vi "Descarga_VFD.vi"(5 "Fabricante":u32, 6 "Modbus":T4, 7 "Iteraciones (In)":u32, 8 "Motor":T6, 9 "I/O":T7, 10 "Referencias":T5, 11 "Instancia Modbus":refnum<class "Modbus Master.lvclass">) -> (0 "Error Modbus":errorcluster, 2 "Iteraciones (Out)":u32)   [LabVIEW 2013]
uses:
  <vilib>/NI/Modbus Library/API/Master/Modbus Master.lvclass
panel:
  in  "Modbus ACS-180":T1
  in  "Modbus VFD-EL":T2
  in  "Modbus ATV 320":T3
  in  "M ACS-180":T1
  in  "M VFD-EL":T2
  in  "M ATV 320":T3
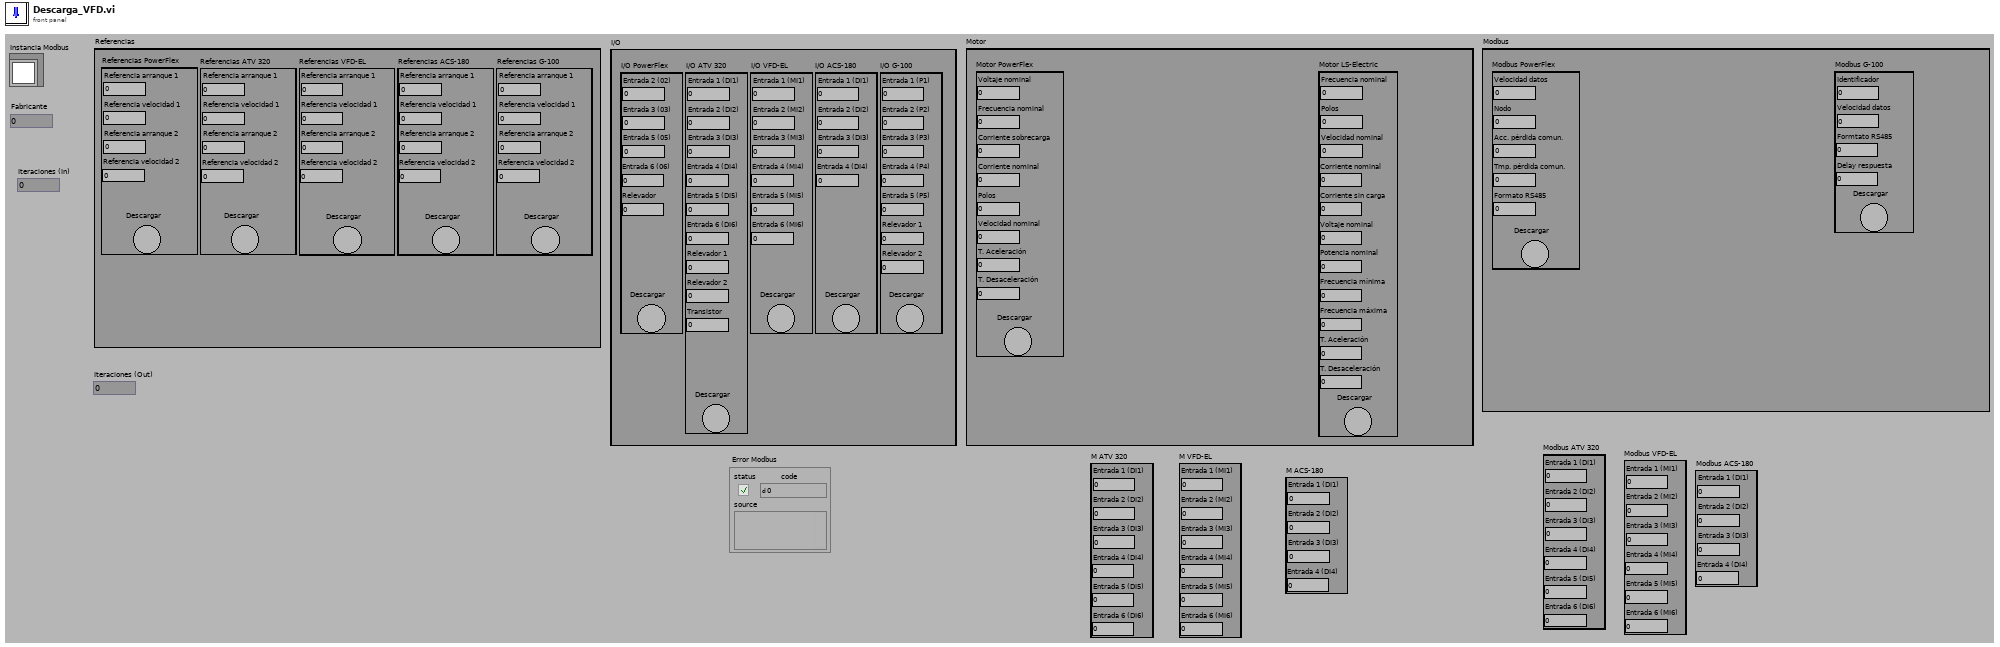
[diagram p1: front panel]
types:
  T1 = cluster{"Entrada 1 (DI1)":u16, "Entrada 2 (DI2)":u16, "Entrada 3 (DI3)":u16, "Entrada 4 (DI4)":u16}
  T2 = cluster{"Entrada 1 (MI1)":u16, "Entrada 2 (MI2)":u16, "Entrada 3 (MI3)":u16, "Entrada 4 (MI4)":u16, "Entrada 5 (MI5)":u16, "Entrada 6 (MI6)":u16}
  T3 = cluster{"Entrada 1 (DI1)":u16, "Entrada 2 (DI2)":u16, "Entrada 3 (DI3)":u16, "Entrada 4 (DI4)":u16, "Entrada 5 (DI5)":u16, "Entrada 6 (DI6)":u16}
  T4 = cluster{"Modbus PowerFlex":cluster{"Velocidad datos":u16, "Nodo":u16, "Acc. pérdida comun.":u16, "Tmp. pérdida comun.":u16, "Formato RS485":u16, "Descargar":bool}, "Modbus G-100":cluster{"Identificador":u16, "Velocidad datos":u16, "Formtato RS485":u16, "Delay respuesta":u16, "Descargar":bool}}
  T5 = cluster{"Referencias PowerFlex":cluster{"Referencia arranque 1":u16, "Referencia velocidad 1":u16, "Referencia arranque 2":u16, "Referencia velocidad 2":u16, "Descargar":bool}, "Referencias ATV 320":cluster{"Referencia arranque 1":u16, "Referencia velocidad 1":u16, "Referencia arranque 2":u16, "Referencia velocidad 2":u16, "Descargar":bool}, "Referencias VFD-EL":cluster{"Referencia arranque 1":u16, "Referencia velocidad 1":u16, "Referencia arranque 2":u16, "Referencia velocidad 2":u16, "Descargar":bool}, "Referencias ACS-180":cluster{"Referencia arranque 1":u16, "Referencia velocidad 1":u16, "Referencia arranque 2":u16, "Referencia velocidad 2":u16, "Descargar":bool}, "Referencias G-100":cluster{"Referencia arranque 1":u16, "Referencia velocidad 1":u16, "Referencia arranque 2":u16, "Referencia velocidad 2":u16, "Descargar":bool}}
  T6 = cluster{"Motor PowerFlex":cluster{"Voltaje nominal":u16, "Frecuencia nominal":u16, "Corriente sobrecarga":dbl, "Corriente nominal":dbl, "Polos":u16, "Velocidad nominal":u16, "T. Aceleración":dbl, "T. Desaceleración":dbl, "Descargar":bool}, "Motor LS-Electric":cluster{"Frecuencia nominal":u16, "Polos":u16, "Velocidad nominal":u16, "Corriente nominal":dbl, "Corriente sin carga":dbl, "Voltaje nominal":u16, "Potencia nominal":u16, "Frecuencia mínima":dbl, "Frecuencia máxima":dbl, "T. Aceleración":dbl, "T. Desaceleración":dbl, "Descargar":bool}}
  T7 = cluster{"I/O PowerFlex":cluster{"Entrada 2 (02)":u16, "Entrada 3 (03)":u16, "Entrada 5 (05)":u16, "Entrada 6 (06)":u16, "Relevador":u16, "Descargar":bool}, "I/O ATV 320":cluster{"Entrada 1 (DI1)":u16, "Entrada 2 (DI2)":u16, "Entrada 3 (DI3)":u16, "Entrada 4 (DI4)":u16, "Entrada 5 (DI5)":u16, "Entrada 6 (DI6)":u16, "Relevador 1":u16, "Relevador 2":u16, "Transistor":u16, "Descargar":bool}, "I/O VFD-EL":cluster{"Entrada 1 (MI1)":u16, "Entrada 2 (MI2)":u16, "Entrada 3 (MI3)":u16, "Entrada 4 (MI4)":u16, "Entrada 5 (MI5)":u16, "Entrada 6 (MI6)":u16, "Descargar":bool}, "I/O ACS-180":cluster{"Entrada 1 (DI1)":u16, "Entrada 2 (DI2)":u16, "Entrada 3 (DI3)":u16, "Entrada 4 (DI4)":u16, "Descargar":bool}, "I/O G-100":cluster{"Entrada 1 (P1)":u16, "Entrada 2 (P2)":u16, "Entrada 3 (P3)":u16, "Entrada 4 (P4)":u16, "Entrada 5 (P5)":u16, "Relevador 1":u16, "Relevador 2":u16, "Descargar":bool}}
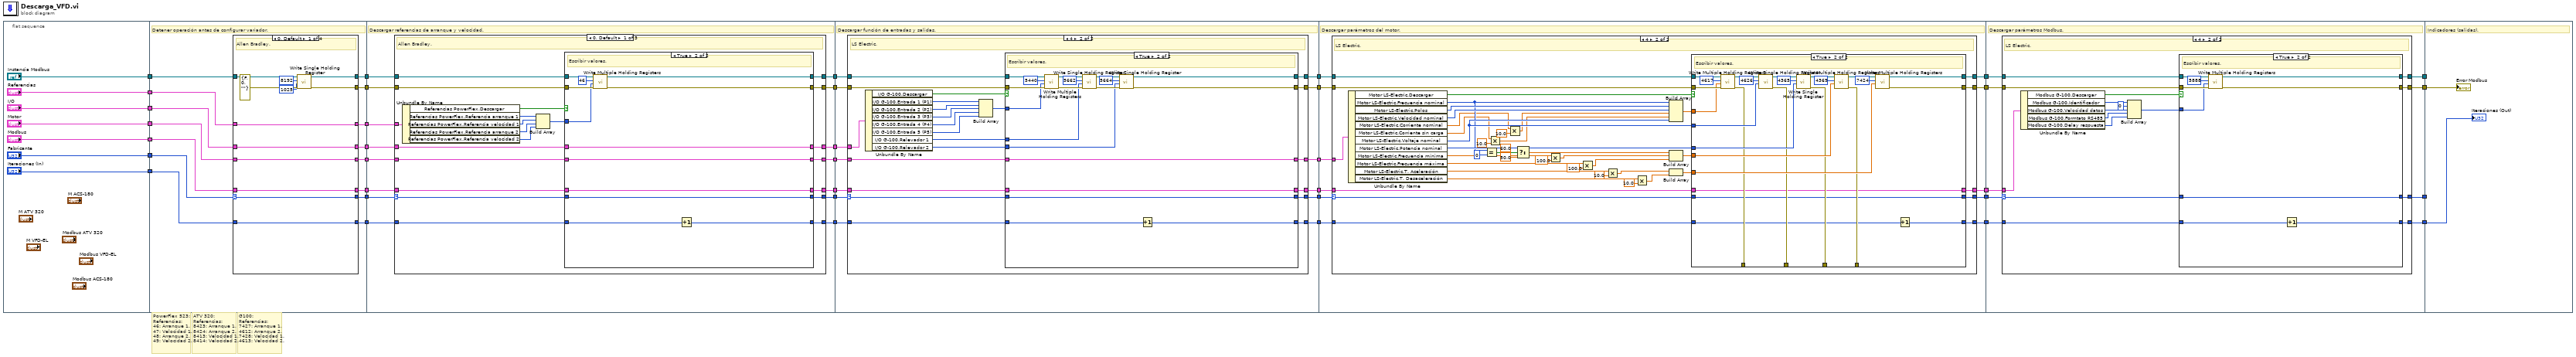
[diagram p0: block diagram]
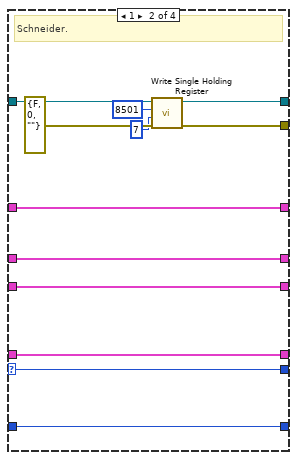
[diagram p2: hidden frame]
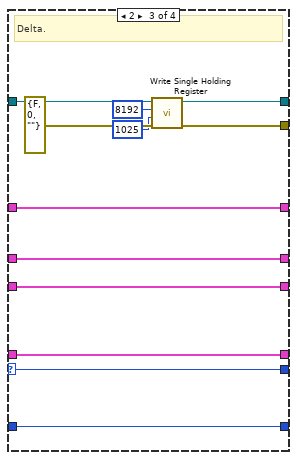
[diagram p3: hidden frame]
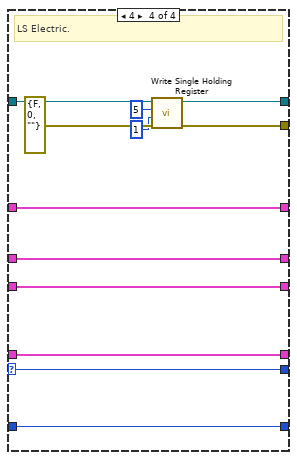
[diagram p4: hidden frame]
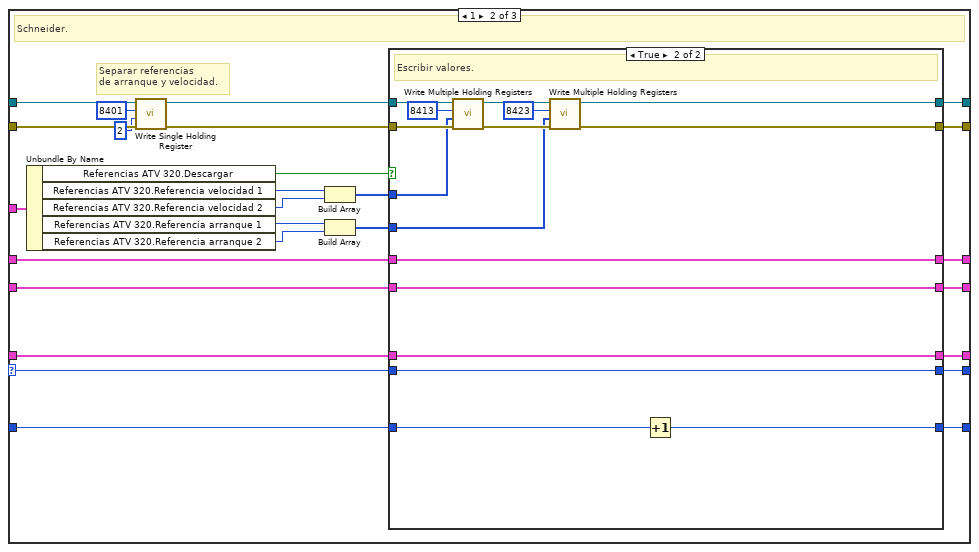
[diagram p6: hidden frame]
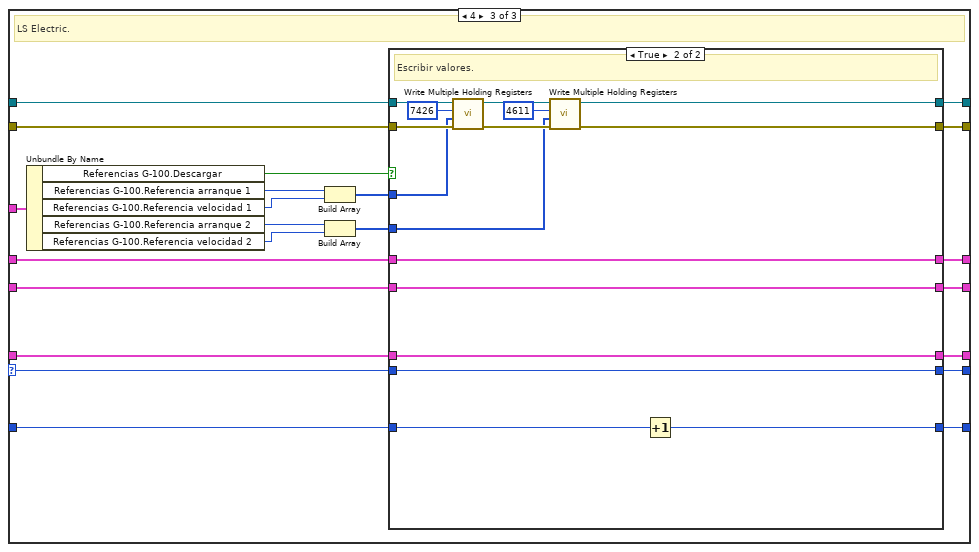
[diagram p8: hidden frame]
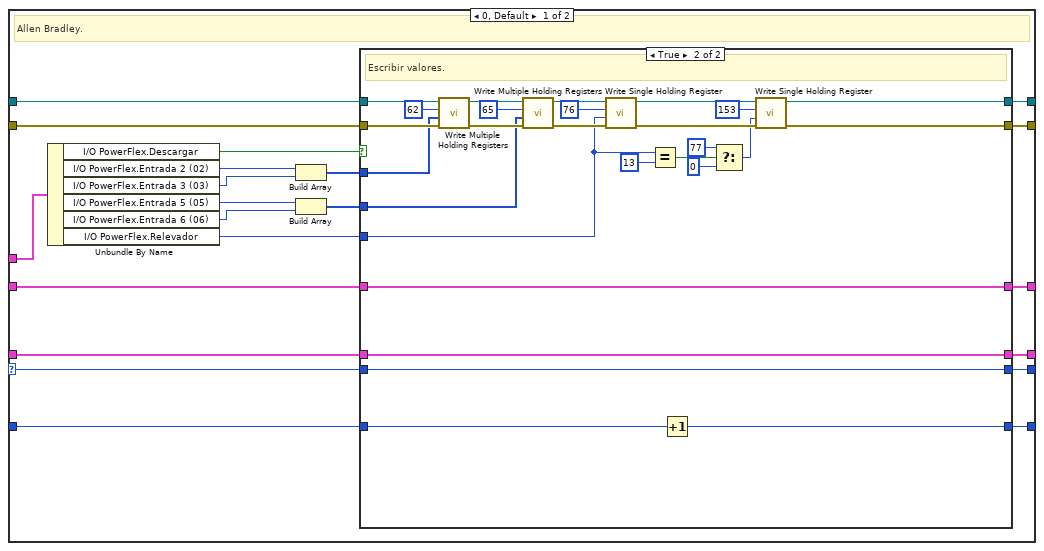
[diagram p10: hidden frame]
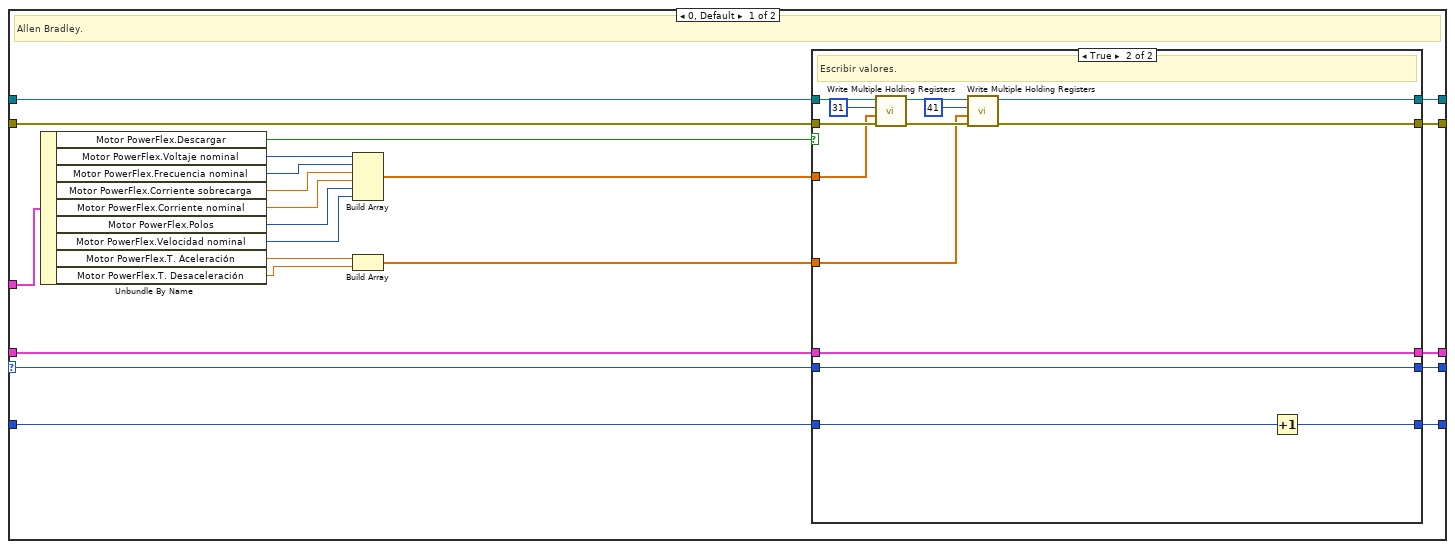
[diagram p13: hidden frame]
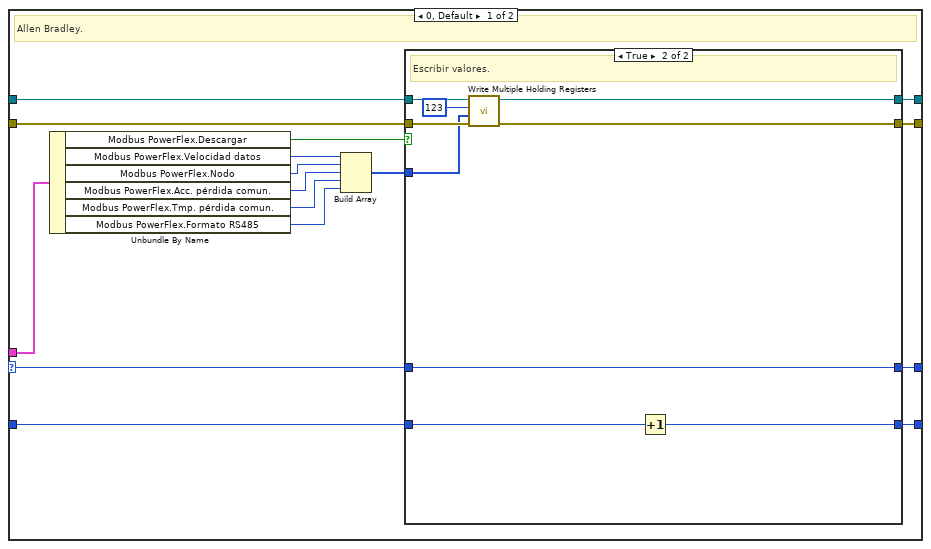
[diagram p16: hidden frame]
diagram:
  # "G100:\nReferencias:\n7427: Arranque 1.\n4612: Arranque 2.\n7428: Velocidad 1.\n4613: Velocidad 2."
  # "ATV 320:\nReferencias:\n8423: Arranque 1.\n8424: Arranque 2.\n8413: Velocidad 1.\n8414: Velocidad 2."
  # "PowerFlex 523:\nReferencias:\n46: Arranque 1.\n47: Velocidad 1.\n48: Arranque 2.\n49: Velocidad 2."
  n1 = flat-sequence {
    tunnel: ["Instancia Modbus"] -> w34
    tunnel: ["Fabricante"] -> w32
    tunnel: ["Referencias"] -> w31
    tunnel: ["I/O"] -> w27
    tunnel: ["Motor"] -> w21
    tunnel: ["Iteraciones (In)"] -> w17
    tunnel: ["Modbus"] -> w13
    tunnel: w34 -> [w59]
    tunnel: [w58] -> w33
    tunnel: w32 -> [w56]
    tunnel: w31 -> [w54]
    tunnel: [w53] -> w30
    tunnel: [w57] -> w29
    tunnel: [w55] -> w28
    tunnel: w27 -> [w52]
    tunnel: [w51] -> w26
    tunnel: w21 -> [w50]
    tunnel: [w49] -> w20
    tunnel: w17 -> [w48]
    tunnel: [w47] -> w16
    tunnel: w13 -> [w46]
    tunnel: [w45] -> w12
    tunnel: w33 -> [w122]
    tunnel: w30 -> [w120]
    tunnel: [w121] -> w37
    tunnel: [w119] -> w36
    tunnel: [w118] -> w35
    tunnel: w29 -> [w117]
    tunnel: w28 -> [w116]
    tunnel: w26 -> [w115]
    tunnel: [w114] -> w25
    tunnel: w20 -> [w113]
    tunnel: [w112] -> w19
    tunnel: w16 -> [w111]
    tunnel: [w110] -> w15
    tunnel: w12 -> [w109]
    tunnel: [w108] -> w11
    tunnel: w37 -> [w268]
    tunnel: w36 -> [w267]
    tunnel: w35 -> [w269]
    tunnel: w25 -> [w266]
    tunnel: [w265] -> w24
    tunnel: [w264] -> w23
    tunnel: [w263] -> w22
    tunnel: w19 -> [w262]
    tunnel: [w261] -> w18
    tunnel: w15 -> [w260]
    tunnel: [w259] -> w14
    tunnel: w11 -> [w258]
    tunnel: [w257] -> w10
    tunnel: w24 -> [w380]
    tunnel: w23 -> [w379]
    tunnel: w22 -> [w381]
    tunnel: w18 -> [w378]
    tunnel: w14 -> [w377]
    tunnel: w10 -> [w376]
    tunnel: [w375] -> w9
    tunnel: [w374] -> w8
    tunnel: [w373] -> w7
    tunnel: [w372] -> w6
    tunnel: [w371] -> w5
    tunnel: w9 -> [w505]
    tunnel: w8 -> [w504]
    tunnel: w7 -> [w501]
    tunnel: w6 -> [w503]
    tunnel: w5 -> [w502]
    tunnel: [w500] -> w4
    tunnel: [w499] -> w3
    tunnel: [w498] -> w2
    tunnel: [w497] -> w1
    tunnel: w4 -> [w565]
    tunnel: w3 -> [_]
    tunnel: w2 -> [w564]
    tunnel: w1 -> [_]
    frame #0 {
    }
    frame #1 {
      # "Detener operación antes de configurar variador."
      n2 = case shown="0, Default" w56 {
        selector: w56 -> [w70 w82 w94 w106]
        tunnel: w59 -> [w67 w79 w91 w103]
        tunnel: [w65 w77 w89 w101] -> w58
        tunnel: [w66 w78 w90 w102] -> w57
        tunnel: [w70 w82 w94 w106] -> w55
        tunnel: w54 -> [w64 w76 w88 w100]
        tunnel: [w64 w76 w88 w100] -> w53
        tunnel: w52 -> [w63 w75 w87 w99]
        tunnel: [w63 w75 w87 w99] -> w51
        tunnel: w50 -> [w62 w74 w86 w98]
        tunnel: [w62 w74 w86 w98] -> w49
        tunnel: w48 -> [w61 w73 w85 w97]
        tunnel: [w61 w73 w85 w97] -> w47
        tunnel: w46 -> [w60 w72 w84 w96]
        tunnel: [w60 w72 w84 w96] -> w45
        frame 0, Default {
          # "Allen Bradley."
          n3 = call-dynamic "Write Single Holding Register.vi"("error in"=errorcluster {"status"=FALSE, "code"=0, "source"=""}, "register to write"=u16 1025, "address"=u16 8192, "Modbus master in"=w67) -> ("error out"=w66:errorcluster, "Modbus master out"=w65:refnum<class "Modbus Master.lvclass">)  [unwired: 6 in]
        }
        frame 1 {
          # "Schneider."
          n4 = call-dynamic "Write Single Holding Register.vi"("error in"=errorcluster {"status"=FALSE, "code"=0, "source"=""}, "register to write"=u16 7, "address"=u16 8501, "Modbus master in"=w79) -> ("error out"=w78:errorcluster, "Modbus master out"=w77:refnum<class "Modbus Master.lvclass">)  [unwired: 6 in]
        }
        frame 2 {
          # "Delta."
          n5 = call-dynamic "Write Single Holding Register.vi"("error in"=errorcluster {"status"=FALSE, "code"=0, "source"=""}, "register to write"=u16 1025, "address"=u16 8192, "Modbus master in"=w91) -> ("error out"=w90:errorcluster, "Modbus master out"=w89:refnum<class "Modbus Master.lvclass">)  [unwired: 6 in]
        }
        frame 4 {
          # "LS Electric."
          n6 = call-dynamic "Write Single Holding Register.vi"("error in"=errorcluster {"status"=FALSE, "code"=0, "source"=""}, "register to write"=u16 1, "address"=u16 5, "Modbus master in"=w103) -> ("error out"=w102:errorcluster, "Modbus master out"=w101:refnum<class "Modbus Master.lvclass">)  [unwired: 6 in]
        }
      }
    }
    frame #2 {
      # "Descargar referencias de arranque y velocidad."
      n7 = case shown="0, Default" w116 {
        selector: w116 -> [w129 w169 w215]
        tunnel: w122 -> [w139 w183 w232]
        tunnel: [w142 w185 w229] -> w121
        tunnel: w120 -> [w141 w186 w230]
        tunnel: [w140 w184 w228] -> w119
        tunnel: [w124 w164 w214] -> w118
        tunnel: w117 -> [w143 w188 w233]
        tunnel: w115 -> [w132 w172 w221]
        tunnel: [w127 w167 w220] -> w114
        tunnel: w113 -> [w131 w171 w219]
        tunnel: [w126 w166 w218] -> w112
        tunnel: w111 -> [w128 w168 w213]
        tunnel: [w123 w163 w212] -> w110
        tunnel: w109 -> [w130 w170 w217]
        tunnel: [w125 w165 w216] -> w108
        frame 0, Default {
          # "Allen Bradley."
          n8 = Unbundle By Name(w141) -> ("Referencias PowerFlex.Descargar"=w133:bool, "Referencias PowerFlex.Referencia arranque 1"=w137:u16, "Referencias PowerFlex.Referencia velocidad 1"=w136:u16, "Referencias PowerFlex.Referencia arranque 2"=w135:u16, "Referencias PowerFlex.Referencia velocidad 2"=w134:u16)
          n9 = Build Array(w137, w136, w135, w134) -> (w138:u16[])
          n10 = case shown="True" w133 {
            tunnel: w143 -> [w149 w162]
            tunnel: [w150 w161] -> w142
            tunnel: [w149 w159] -> w140
            tunnel: w139 -> [w150 w158]
            tunnel: w138 -> [_ w157]
            tunnel: w132 -> [w148 w156]
            tunnel: w131 -> [w147 w155]
            tunnel: w130 -> [w146 w154]
            tunnel: w129 -> [w145 w153]
            tunnel: w128 -> [w144 w152]
            tunnel: [w148 w156] -> w127
            tunnel: [w147 w155] -> w126
            tunnel: [w146 w154] -> w125
            tunnel: [w145 w153] -> w124
            tunnel: [w144 w151] -> w123
            frame False {
              # "Nada."
            }
            frame True {
              # "Escribir valores."
              n11 = call-dynamic "Write Multiple Holding Registers.vi"("error in"=w162, "registers to write"=w157, "starting address"=u16 46, "Modbus master in"=w158) -> ("error out"=w159:errorcluster, "Modbus master out"=w161:refnum<class "Modbus Master.lvclass">)  [unwired: 6 in]
              n12 = Increment(x=w152) -> (x+1=w151:u32)
            }
          }
        }
        frame 1 {
          # "Separar referencias\nde arranque y velocidad."
          # "Schneider."
          n13 = Unbundle By Name(w186) -> ("Referencias ATV 320.Descargar"=w177:bool, "Referencias ATV 320.Referencia velocidad 1"=w176:u16, "Referencias ATV 320.Referencia velocidad 2"=w175:u16, "Referencias ATV 320.Referencia arranque 1"=w174:u16, "Referencias ATV 320.Referencia arranque 2"=w173:u16)
          n14 = call-dynamic "Write Single Holding Register.vi"("error in"=w188, "register to write"=u16 2, "address"=u16 8401, "Modbus master in"=w183) -> ("error out"=w187:errorcluster, "Modbus master out"=w182:refnum<class "Modbus Master.lvclass">)  [unwired: 6 in]
          n15 = Build Array(w176, w175) -> (w179:u16[])
          n16 = Build Array(w174, w173) -> (w178:u16[])
          n17 = case shown="True" w177 {
            tunnel: w187 -> [w194 w211]
            tunnel: [w195 w207] -> w185
            tunnel: [w194 w206] -> w184
            tunnel: w182 -> [w195 w204]
            tunnel: w179 -> [_ w203]
            tunnel: w178 -> [_ w202]
            tunnel: w172 -> [w193 w201]
            tunnel: w171 -> [w192 w200]
            tunnel: w170 -> [w191 w199]
            tunnel: w169 -> [w190 w198]
            tunnel: w168 -> [w189 w197]
            tunnel: [w193 w201] -> w167
            tunnel: [w192 w200] -> w166
            tunnel: [w191 w199] -> w165
            tunnel: [w190 w198] -> w164
            tunnel: [w189 w196] -> w163
            frame False {
              # "Nada."
            }
            frame True {
              # "Escribir valores."
              n18 = call-dynamic "Write Multiple Holding Registers.vi"("error in"=w211, "registers to write"=w203, "starting address"=u16 8413, "Modbus master in"=w204) -> ("error out"=w205:errorcluster, "Modbus master out"=w208:refnum<class "Modbus Master.lvclass">)  [unwired: 6 in]
              n19 = call-dynamic "Write Multiple Holding Registers.vi"("error in"=w205, "registers to write"=w202, "starting address"=u16 8423, "Modbus master in"=w208) -> ("error out"=w206:errorcluster, "Modbus master out"=w207:refnum<class "Modbus Master.lvclass">)  [unwired: 6 in]
              n20 = Increment(x=w197) -> (x+1=w196:u32)
            }
          }
        }
        frame 4 {
          # "LS Electric."
          n21 = Unbundle By Name(w230) -> ("Referencias G-100.Descargar"=w226:bool, "Referencias G-100.Referencia arranque 1"=w225:u16, "Referencias G-100.Referencia velocidad 1"=w224:u16, "Referencias G-100.Referencia arranque 2"=w223:u16, "Referencias G-100.Referencia velocidad 2"=w222:u16)
          n22 = Build Array(w225, w224) -> (w231:u16[])
          n23 = Build Array(w223, w222) -> (w227:u16[])
          n24 = case shown="True" w226 {
            tunnel: w233 -> [w239 w256]
            tunnel: w232 -> [w240 w255]
            tunnel: w231 -> [_ w253]
            tunnel: [w240 w250] -> w229
            tunnel: [w239 w249] -> w228
            tunnel: w227 -> [_ w247]
            tunnel: w221 -> [w238 w246]
            tunnel: [w238 w246] -> w220
            tunnel: w219 -> [w237 w245]
            tunnel: [w237 w245] -> w218
            tunnel: w217 -> [w236 w244]
            tunnel: [w236 w244] -> w216
            tunnel: [w235 w243] -> w214
            tunnel: w215 -> [w235 w243]
            tunnel: w213 -> [w234 w242]
            tunnel: [w234 w241] -> w212
            frame False {
              # "Nada."
            }
            frame True {
              # "Escribir valores."
              n25 = call-dynamic "Write Multiple Holding Registers.vi"("error in"=w256, "registers to write"=w253, "starting address"=u16 7426, "Modbus master in"=w255) -> ("error out"=w248:errorcluster, "Modbus master out"=w251:refnum<class "Modbus Master.lvclass">)  [unwired: 6 in]
              n26 = call-dynamic "Write Multiple Holding Registers.vi"("error in"=w248, "registers to write"=w247, "starting address"=u16 4611, "Modbus master in"=w251) -> ("error out"=w249:errorcluster, "Modbus master out"=w250:refnum<class "Modbus Master.lvclass">)  [unwired: 6 in]
              n27 = Increment(x=w242) -> (x+1=w241:u32)
            }
          }
        }
      }
    }
    frame #3 {
      # "Descargar función de entradas y salidas."
      n28 = case shown="4" w269 {
        selector: w269 -> [w275 w329]
        tunnel: w268 -> [w288 w342]
        tunnel: [w271 w325] -> w263
        tunnel: w267 -> [w289 w343]
        tunnel: w266 -> [w290 w344]
        tunnel: [w285 w340] -> w265
        tunnel: [w284 w339] -> w264
        tunnel: w262 -> [w277 w331]
        tunnel: [w273 w327] -> w261
        tunnel: w260 -> [w274 w328]
        tunnel: [w270 w324] -> w259
        tunnel: w258 -> [w276 w330]
        tunnel: [w272 w326] -> w257
        frame 0, Default {
          # "Allen Bradley."
          n29 = Unbundle By Name(w290) -> ("I/O PowerFlex.Descargar"=w278:bool, "I/O PowerFlex.Entrada 2 (02)"=w282:u16, "I/O PowerFlex.Entrada 3 (03)"=w281:u16, "I/O PowerFlex.Entrada 5 (05)"=w280:u16, "I/O PowerFlex.Entrada 6 (06)"=w279:u16, "I/O PowerFlex.Relevador"=w283:u16)
          n30 = Build Array(w282, w281) -> (w287:u16[])
          n31 = Build Array(w280, w279) -> (w286:u16[])
          n32 = case shown="True" w278 {
            tunnel: w289 -> [w295 w322]
            tunnel: w288 -> [w296 w321]
            tunnel: w287 -> [_ w319]
            tunnel: w286 -> [_ w315]
            tunnel: [w296 w304] -> w285
            tunnel: [w295 w303] -> w284
            tunnel: w283 -> [_ w302]
            tunnel: w277 -> [w294 w301]
            tunnel: w276 -> [w293 w300]
            tunnel: w275 -> [w292 w299]
            tunnel: w274 -> [w291 w298]
            tunnel: [w294 w301] -> w273
            tunnel: [w293 w300] -> w272
            tunnel: [w292 w299] -> w271
            tunnel: [w291 w297] -> w270
            frame False {
              # "Nada."
            }
            frame True {
              # "Escribir valores."
              n33 = call-dynamic "Write Multiple Holding Registers.vi"("error in"=w322, "registers to write"=w319, "starting address"=u16 62, "Modbus master in"=w321) -> ("error out"=w316:errorcluster, "Modbus master out"=w317:refnum<class "Modbus Master.lvclass">)  [unwired: 6 in]
              n34 = call-dynamic "Write Multiple Holding Registers.vi"("error in"=w316, "registers to write"=w315, "starting address"=u16 65, "Modbus master in"=w317) -> ("error out"=w323:errorcluster, "Modbus master out"=w313:refnum<class "Modbus Master.lvclass">)  [unwired: 6 in]
              n35 = call-dynamic "Write Single Holding Register.vi"("error in"=w323, "register to write"=w302, "address"=u16 76 ("starting address"), "Modbus master in"=w313) -> ("error out"=w311:errorcluster, "Modbus master out"=w310:refnum<class "Modbus Master.lvclass">)  [unwired: 6 in]
              n36 = Equal?(x=w302, y=u16 13) -> (x = y?=w308:bool)
              n37 = Increment(x=w298) -> (x+1=w297:u32)
              n38 = Select(t=u16 77 ("register to write"), s=w308, f=u16 0 ("register to write")) -> (s? t:f=w305:u16)
              n39 = call-dynamic "Write Single Holding Register.vi"("error in"=w311, "register to write"=w305, "address"=u16 153 ("starting address"), "Modbus master in"=w310) -> ("error out"=w303:errorcluster, "Modbus master out"=w304:refnum<class "Modbus Master.lvclass">)  [unwired: 6 in]
            }
          }
        }
        frame 4 {
          # "LS Electric."
          n40 = Unbundle By Name(w344) -> ("I/O G-100.Descargar"=w335:bool, "I/O G-100.Entrada 1 (P1)"=w333:u16, "I/O G-100.Entrada 2 (P2)"=w332:u16, "I/O G-100.Entrada 3 (P3)"=w338:u16, "I/O G-100.Entrada 4 (P4)"=w337:u16, "I/O G-100.Entrada 5 (P5)"=w336:u16, "I/O G-100.Relevador 1"=w345:u16, "I/O G-100.Relevador 2"=w334:u16)
          n41 = Build Array(w333, w332, w338, w337, w336) -> (w341:u16[])
          n42 = case shown="True" w335 {
            tunnel: w345 -> [_ w358]
            tunnel: w343 -> [w350 w368]
            tunnel: w342 -> [w351 w367]
            tunnel: w341 -> [_ w365]
            tunnel: [w351 w362] -> w340
            tunnel: [w350 w361] -> w339
            tunnel: w334 -> [_ w357]
            tunnel: w331 -> [w349 w356]
            tunnel: w330 -> [w348 w355]
            tunnel: w329 -> [w347 w354]
            tunnel: w328 -> [w346 w353]
            tunnel: [w349 w356] -> w327
            tunnel: [w348 w355] -> w326
            tunnel: [w347 w354] -> w325
            tunnel: [w346 w352] -> w324
            frame False {
              # "Nada."
            }
            frame True {
              # "Escribir valores."
              n43 = call-dynamic "Write Multiple Holding Registers.vi"("error in"=w368, "registers to write"=w365, "starting address"=u16 5440, "Modbus master in"=w367) -> ("error out"=w370:errorcluster, "Modbus master out"=w364:refnum<class "Modbus Master.lvclass">)  [unwired: 6 in]
              n44 = call-dynamic "Write Single Holding Register.vi"("error in"=w370, "register to write"=w358, "address"=u16 5662, "Modbus master in"=w364) -> ("error out"=w369:errorcluster, "Modbus master out"=w363:refnum<class "Modbus Master.lvclass">)  [unwired: 6 in]
              n45 = call-dynamic "Write Single Holding Register.vi"("error in"=w369, "register to write"=w357, "address"=u16 5664, "Modbus master in"=w363) -> ("error out"=w361:errorcluster, "Modbus master out"=w362:refnum<class "Modbus Master.lvclass">)  [unwired: 6 in]
              n46 = Increment(x=w353) -> (x+1=w352:u32)
            }
          }
        }
      }
    }
    frame #4 {
      # "Descargar parámetros del motor."
      n47 = case shown="4" w381 {
        selector: w381 -> [w386 w427]
        tunnel: w380 -> [w400 w462]
        tunnel: [w383 w425] -> w373
        tunnel: w379 -> [w401 w463]
        tunnel: w378 -> [w402 w464]
        tunnel: [w397 w460] -> w375
        tunnel: [w398 w459] -> w374
        tunnel: w377 -> [w385 w426]
        tunnel: w376 -> [w387 w428]
        tunnel: [w384 w423] -> w372
        tunnel: [w382 w424] -> w371
        frame 0, Default {
          # "Allen Bradley."
          n48 = Unbundle By Name(w402) -> ("Motor PowerFlex.Descargar"=w390:bool, "Motor PowerFlex.Voltaje nominal"=w395:u16, "Motor PowerFlex.Frecuencia nominal"=w388:u16, "Motor PowerFlex.Corriente sobrecarga"=w394:dbl, "Motor PowerFlex.Corriente nominal"=w393:dbl, "Motor PowerFlex.Polos"=w392:u16, "Motor PowerFlex.Velocidad nominal"=w391:u16, "Motor PowerFlex.T. Aceleración"=w396:dbl, "Motor PowerFlex.T. Desaceleración"=w389:dbl)
          n49 = Build Array(w395, w388, w394, w393, w392, w391) -> (w399:dbl[])
          n50 = Build Array(w396, w389) -> (w403:dbl[])
          n51 = case shown="True" w390 {
            tunnel: w403 -> [_ w421]
            tunnel: w401 -> [w407 w420]
            tunnel: w400 -> [w408 w419]
            tunnel: w399 -> [_ w417]
            tunnel: [w407 w414] -> w398
            tunnel: [w408 w413] -> w397
            tunnel: w387 -> [w406 w412]
            tunnel: w386 -> [w405 w411]
            tunnel: w385 -> [w404 w410]
            tunnel: [w406 w412] -> w384
            tunnel: [w405 w411] -> w383
            tunnel: [w404 w409] -> w382
            frame False {
              # "Nada."
            }
            frame True {
              # "Escribir valores."
              n52 = call-dynamic "Write Multiple Holding Registers.vi"("error in"=w420, "registers to write"=w417, "starting address"=u16 31, "Modbus master in"=w419) -> ("error out"=w422:errorcluster, "Modbus master out"=w415:refnum<class "Modbus Master.lvclass">)  [unwired: 6 in]
              n53 = call-dynamic "Write Multiple Holding Registers.vi"("error in"=w422, "registers to write"=w421, "starting address"=u16 41, "Modbus master in"=w415) -> ("error out"=w414:errorcluster, "Modbus master out"=w413:refnum<class "Modbus Master.lvclass">)  [unwired: 6 in]
              n54 = Increment(x=w410) -> (x+1=w409:u32)
            }
          }
        }
        frame 4 {
          # "LS Electric."
          n55 = Unbundle By Name(w464) -> ("Motor LS-Electric.Descargar"=w458:bool, "Motor LS-Electric.Frecuencia nominal"=w450:u16, "Motor LS-Electric.Polos"=w452:u16, "Motor LS-Electric.Velocidad nominal"=w457:u16, "Motor LS-Electric.Corriente nominal"=w446:dbl, "Motor LS-Electric.Corriente sin carga"=w442:dbl, "Motor LS-Electric.Voltaje nominal"=w455:u16, "Motor LS-Electric.Potencia nominal"=w456:u16, "Motor LS-Electric.Frecuencia mínima"=w438:dbl, "Motor LS-Electric.Frecuencia máxima"=w436:dbl, "Motor LS-Electric.T. Aceleración"=w433:dbl, "Motor LS-Electric.T. Desaceleración"=w430:dbl)
          n56 = Equal?(x=w450, y=u16 0) -> (x = y?=w449:bool)
          n57 = Multiply(x=w442, y=10.0) -> (x*y=w441:dbl)
          n58 = Multiply(x=w446, y=10.0) -> (x*y=w444:dbl)
          n59 = Select(t=60.0, s=w449, f=50.0) -> (s? t:f=w465:dbl)
          n60 = Multiply(x=w438, y=100.0) -> (x*y=w437:dbl)
          n61 = Multiply(x=w436, y=100.0) -> (x*y=w435:dbl)
          n62 = Multiply(x=w433, y=10.0) -> (x*y=w432:dbl)
          n63 = Multiply(x=w430, y=10.0) -> (x*y=w429:dbl)
          n64 = Build Array(w450, w452, w457, w444, w441, w455) -> (w461:dbl[])
          n65 = Build Array(w465, w437, w435) -> (w454:dbl[])
          n66 = Build Array(w432, w429) -> (w453:dbl[])
          n67 = case shown="True" w458 {
            tunnel: w463 -> [w469 w495]
            tunnel: w462 -> [w470 w494]
            tunnel: w461 -> [_ w492]
            tunnel: [w470 w481] -> w460
            tunnel: [w469 w480] -> w459
            tunnel: w456 -> [_ w484]
            tunnel: w455 -> [_ w485]
            tunnel: w454 -> [_ w496]
            tunnel: w453 -> [_ w479]
            tunnel: [_ w478] -> _
            tunnel: [_ w477] -> _
            tunnel: [_ w476] -> _
            tunnel: [_ w475] -> _
            tunnel: w428 -> [w468 w471]
            tunnel: w427 -> [w467 w474]
            tunnel: w426 -> [w466 w473]
            tunnel: [w467 w474] -> w425
            tunnel: [w466 w472] -> w424
            tunnel: [w468 w471] -> w423
            frame False {
              # "Nada."
            }
            frame True {
              # "Escribir valores."
              n68 = call-dynamic "Write Multiple Holding Registers.vi"("error in"=w495, "registers to write"=w492, "starting address"=u16 4617, "Modbus master in"=w494) -> ("error out"=w478:errorcluster, "Modbus master out"=w487:refnum<class "Modbus Master.lvclass">)  [unwired: 6 in]
              n69 = call-dynamic "Write Single Holding Register.vi"("register to write"=w485, "address"=u16 4626, "Modbus master in"=w487) -> ("error out"=w477:errorcluster, "Modbus master out"=w486:refnum<class "Modbus Master.lvclass">)  [unwired: 7 in]
              n70 = call-dynamic "Write Single Holding Register.vi"("register to write"=w484, "address"=u16 4365, "Modbus master in"=w486) -> ("error out"=w476:errorcluster, "Modbus master out"=w491:refnum<class "Modbus Master.lvclass">)  [unwired: 7 in]
              n71 = call-dynamic "Write Multiple Holding Registers.vi"("registers to write"=w496, "starting address"=u16 4369 ("address"), "Modbus master in"=w491) -> ("error out"=w475:errorcluster, "Modbus master out"=w482:refnum<class "Modbus Master.lvclass">)  [unwired: 7 in]
              n72 = call-dynamic "Write Multiple Holding Registers.vi"("registers to write"=w479, "starting address"=u16 7424 ("address"), "Modbus master in"=w482) -> ("error out"=w480:errorcluster, "Modbus master out"=w481:refnum<class "Modbus Master.lvclass">)  [unwired: 7 in]
              n73 = Increment(x=w473) -> (x+1=w472:u32)
            }
          }
        }
      }
    }
    frame #5 {
      # "Descargar parámetros Modbus."
      n74 = case shown="4" w501 {
        selector: w501 -> [w509 w538]
        tunnel: w505 -> [w520 w548]
        tunnel: [w507 w536] -> w497
        tunnel: w504 -> [w521 w549]
        tunnel: [w517 w546] -> w499
        tunnel: [w518 w545] -> w498
        tunnel: w502 -> [w508 w537]
        tunnel: w503 -> [w513 w543]
        tunnel: [w506 w535] -> w500
        frame 0, Default {
          # "Allen Bradley."
          n75 = Unbundle By Name(w513) -> ("Modbus PowerFlex.Descargar"=w514:bool, "Modbus PowerFlex.Velocidad datos"=w512:u16, "Modbus PowerFlex.Nodo"=w511:u16, "Modbus PowerFlex.Acc. pérdida comun."=w510:u16, "Modbus PowerFlex.Tmp. pérdida comun."=w516:u16, "Modbus PowerFlex.Formato RS485"=w515:u16)
          n76 = Build Array(w512, w511, w510, w516, w515) -> (w519:u16[])
          n77 = case shown="True" w514 {
            tunnel: w521 -> [w524 w534]
            tunnel: w520 -> [w525 w533]
            tunnel: w519 -> [_ w531]
            tunnel: [w524 w529] -> w518
            tunnel: [w525 w530] -> w517
            tunnel: w509 -> [w523 w528]
            tunnel: w508 -> [w522 w527]
            tunnel: [w523 w528] -> w507
            tunnel: [w522 w526] -> w506
            frame False {
              # "Nada."
            }
            frame True {
              # "Escribir valores."
              n78 = call-dynamic "Write Multiple Holding Registers.vi"("error in"=w534, "registers to write"=w531, "starting address"=u16 123, "Modbus master in"=w533) -> ("error out"=w529:errorcluster, "Modbus master out"=w530:refnum<class "Modbus Master.lvclass">)  [unwired: 6 in]
              n79 = Increment(x=w527) -> (x+1=w526:u32)
            }
          }
        }
        frame 4 {
          # "LS Electric."
          n80 = Unbundle By Name(w543) -> ("Modbus G-100.Descargar"=w544:bool, "Modbus G-100.Identificador"=w550:u16, "Modbus G-100.Velocidad datos"=w541:u16, "Modbus G-100.Formtato RS485"=w540:u16, "Modbus G-100.Delay respuesta"=w539:u16)
          n81 = Build Array(w550, u16 0 ("element"), w541, w540, w539) -> (w547:u16[])
          n82 = case shown="True" w544 {
            tunnel: w549 -> [w553 w563]
            tunnel: w548 -> [w554 w562]
            tunnel: w547 -> [_ w560]
            tunnel: [w554 w559] -> w546
            tunnel: [w553 w558] -> w545
            tunnel: w538 -> [w552 w557]
            tunnel: w537 -> [w551 w556]
            tunnel: [w552 w557] -> w536
            tunnel: [w551 w555] -> w535
            frame False {
              # "Nada."
            }
            frame True {
              # "Escribir valores."
              n83 = call-dynamic "Write Multiple Holding Registers.vi"("error in"=w563, "registers to write"=w560, "starting address"=u16 5888, "Modbus master in"=w562) -> ("error out"=w558:errorcluster, "Modbus master out"=w559:refnum<class "Modbus Master.lvclass">)  [unwired: 6 in]
              n84 = Increment(x=w556) -> (x+1=w555:u32)
            }
          }
        }
      }
    }
    frame #6 {
      # "Indicadores (salidas)."
      "Iteraciones (Out)" <- w565
      "Error Modbus" <- w564
    }
  }
